vi "IT8900A-E Series Run List File.vi"() -> ()   [LabVIEW 2015]
uses:
  <instrlib>/IT8900/IT8900A-E.lvlib
panel:
  in  "Trigger Source 0:BUS":u16(ring) items=["BUS", "External", "HOLD", "Manual", "Timer"]
  in  "Save Type ( 0 : Save)":u16(ring) caption="Save Type" items=["Save", "RCL"]
  in  "?":bool
  in  "List Number (1)":i32=1 min=1 max=7 format="%#_0f"
  out "Current":dbl
  out "Voltage":dbl format="%_6f"
  in  "Serial Configuration":cluster{"Baud Rate":u32}={"Baud Rate"=9600} {"Baud Rate" items=["300"=300, "600"=600, "1200"=1200, "2400"=2400, "4800"=4800, "9600"=9600, "19200"=19200]}
  in  "VISA resource name":refnum<visa-resource-name>
  # "V"
  # "A"
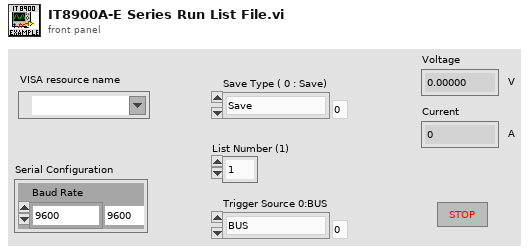
[diagram p1: front panel]
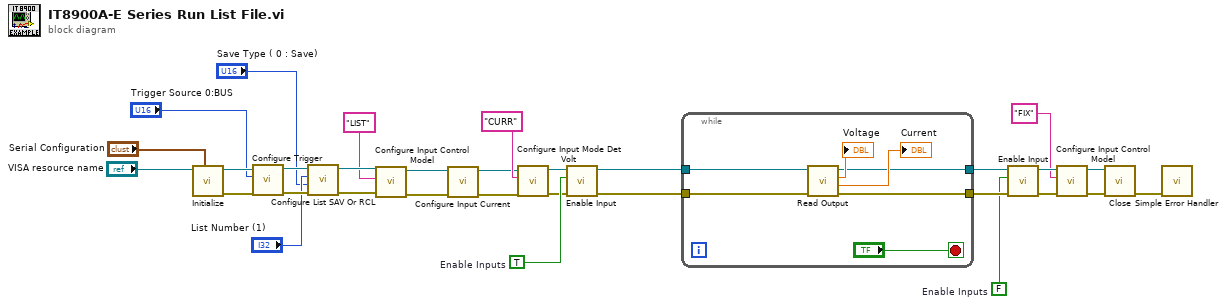
[diagram p0: block diagram]
diagram:
  w16 = FALSE  # Enable Inputs
  w24 = TRUE  # Enable Inputs
  n1 = call <instrlib>:"Initialize.vi"("Serial Configuration"="Serial Configuration", "VISA resource name"="VISA resource name") -> ("error out"=w29:errorcluster, "VISA resource name out"=w28:refnum<visa-resource-name>)  [unwired: 8 in]
  n2 = call <instrlib>:"Configure Trigger.vi"("error in (no error)"=w29, "Trigger Source 0:BUS"="Trigger Source 0:BUS", "VISA resource name"=w28) -> ("error out"=w27:errorcluster, "VISA resource name out"=w26:refnum<visa-resource-name>)  [unwired: 7 in]
  n3 = call <instrlib>:"Configure List SAV Or RCL.vi"("error in (no error)"=w27, "Save Type ( 0 : Save)"="Save Type ( 0 : Save)", "File Add ( 1 - 5 )"="List Number (1)", "VISA resource name"=w26) -> ("error out"=w12:errorcluster, "VISA resource name out"=w13:refnum<visa-resource-name>)  [unwired: 6 in]
  n4 = call <instrlib>:"Configure Input Control Model.vi"("error in (no error)"=w12, "Model"="LIST", "VISA resource name"=w13) -> ("error out"=w4:errorcluster, "VISA resource name out"=w6:refnum<visa-resource-name>)  [unwired: 7 in]
  n5 = call <instrlib>:"Configure Input Current.vi"("error in (no error)"=w4, "VISA resource name"=w6) -> ("error out"=w3:errorcluster, "VISA resource name out"=w5:refnum<visa-resource-name>)  [unwired: 8 in]
  n6 = call <instrlib>:"Configure Input Mode Det Volt.vi"("error in (no error)"=w3, "Type"="CURR", "VISA resource name"=w5) -> ("error out"=w8:errorcluster, "VISA resource name out"=w9:refnum<visa-resource-name>)  [unwired: 7 in]
  n7 = call <instrlib>:"Enable Input.vi"("error in (no error)"=w8, "Enable Input"=w24, "VISA resource name"=w9) -> ("error out"=w14:errorcluster, "VISA resource name out"=w15:refnum<visa-resource-name>)  [unwired: 7 in]
  n8 = while {
    tunnel: [w35] -> w23
    tunnel: [w34] -> w22
    tunnel: w15 -> [w33]
    tunnel: w14 -> [w32]
    stop <- "?" stop-if-true
    n9 = call <instrlib>:"Read Output.vi"("error in (no error)"=w32, "VISA resource name"=w33) -> ("error out"=w34:errorcluster, "Actual Current Level (A)"=→"Current":dbl, "Actual Voltage Level (V)"=→"Voltage":dbl, "VISA resource name out"=w35:refnum<visa-resource-name>)  [unwired: 6 in]
  }
  n10 = call <instrlib>:"Enable Input.vi"("error in (no error)"=w22, "Enable Input"=w16, "VISA resource name"=w23) -> ("error out"=w21:errorcluster, "VISA resource name out"=w20:refnum<visa-resource-name>)  [unwired: 7 in]
  n11 = call <instrlib>:"Configure Input Control Model.vi"("error in (no error)"=w21, "Model"="FIX", "VISA resource name"=w20) -> ("error out"=w19:errorcluster, "VISA resource name out"=w18:refnum<visa-resource-name>)  [unwired: 7 in]
  n12 = call <instrlib>:"Close.vi"("error in (no error)"=w19, "VISA resource name"=w18) -> ("error out"=w17:errorcluster)  [unwired: 9 in]
  n13 = call <vilib>:"Simple Error Handler.vi"("error in (no error)"=w17) -> ()  [unwired: 4 in, 5 out]
